vi "niScope Get Physical Cards.vi"(8 "error in":errorcluster, 11 "niScope in":T1={"channel cfg"=[], "sessions"=[], "multi cards"=FALSE, "channels"=0, "type"=enum."n/a", "memory [B/chn]"=0, "ext. clock [Hz]"=0.0, "samples count"=0, "use streaming"=FALSE, "proc setup"={"packet size [smpl]"=0, "current timeout [s]"=0.0, "blk2blk timeout [s]"=0.0, "event time"=timestamp(0 s since 1904-01-01), "temp sampl T [s]"=0.0, "data queue"=refnum, "stop notifier"=refnum, "proc ref"=refnum}, "sample width [B]"=0, "ranges [V]"=[], "trigger setup"={"coupling"=1, "level [V]"=0.0, "slope"=0, "mode"=enum."Immediate"}, "fs [Hz]"=0.0, "bitres [bit]"=0, "clock source"=enum."VAL_NO_SOURCE"} {"trigger setup"."level [V]" format="%.2f"; "trigger setup"."coupling" items=["AC"=0, "DC"=1, "HF Reject"=3, "LF Reject"=4, "AC Plus HF Reject"=1001]; "channel cfg"."Range [Vpk]" min=0.0; "channel cfg"."Channel" min=0}) -> (0 "error out":errorcluster, 2 "card list":T12[](array[typedef]), 3 "niScope out":T1={"channel cfg"=[], "sessions"=[], "multi cards"=FALSE, "channels"=0, "type"=enum."n/a", "memory [B/chn]"=0, "ext. clock [Hz]"=0.0, "samples count"=0, "use streaming"=FALSE, "proc setup"={"packet size [smpl]"=0, "current timeout [s]"=0.0, "blk2blk timeout [s]"=0.0, "event time"=timestamp(0 s since 1904-01-01), "temp sampl T [s]"=0.0, "data queue"=refnum, "stop notifier"=refnum, "proc ref"=refnum}, "sample width [B]"=0, "ranges [V]"=[], "trigger setup"={"coupling"=1, "level [V]"=0.0, "slope"=0, "mode"=enum."Immediate"}, "fs [Hz]"=0.0, "bitres [bit]"=0, "clock source"=enum."VAL_NO_SOURCE"} {"trigger setup"."level [V]" format="%.2f"; "trigger setup"."coupling" items=["AC"=0, "DC"=1, "HF Reject"=3, "LF Reject"=4, "AC Plus HF Reject"=1001]; "channel cfg"."Range [Vpk]" min=0.0; "channel cfg"."Channel" min=0})   [LabVIEW 2013, in "niScope Virtual Digitizer.lvlib"]
doc: "Scans through virtual channels list and builds list of physical channels for each unique address (device)."
uses:
  niScope Physical Cards.ctl
  niScope Session.ctl
  niScope Virtual Channel Config.ctl
  niScope Virtual Channel Mode.ctl
  niScope Virtual Channel Input Z.ctl
  niScope Virtual Channel Coupling.ctl
  niScope Type.ctl
  niScope Digitizing Process Options.ctl
  niScope Data Packet.ctl
  niScope Trigger Setup.ctl
  <instrlib>/niScope/Controls/niScope trigger coupling.ctl
  <instrlib>/niScope/Controls/niScope trigger slope.ctl
  niScope Reference Clock.ctl
  <vilib>/Utility/error.llb/Error Cluster From Error Code.vi
  <vilib>/ErrorRing/Error Ring.xnode
  niScope Virtual Digitizer.lvlib
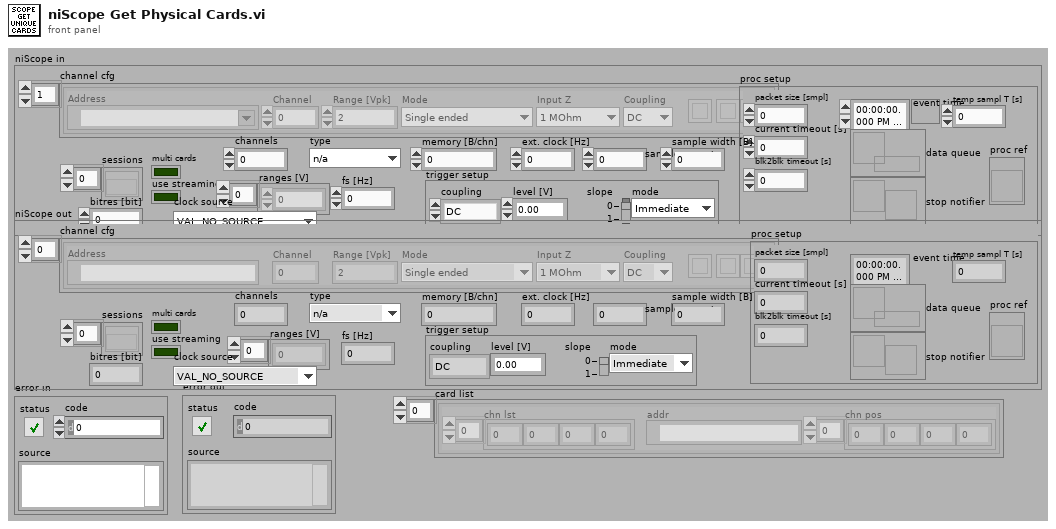
[diagram p1: front panel]
types:
  T1 = typedef "niScope Virtual Digitizer.lvlib/niScope Session.ctl" = cluster{"channel cfg":T2[], "sessions":refnum<k20>[], "multi cards":bool, "channels":i32, "type":T6, "memory [B/chn]":i32, "ext. clock [Hz]":dbl, "samples count":i64, "use streaming":bool, "proc setup":T7, "sample width [B]":i32, "ranges [V]":dbl[], "trigger setup":T8, "fs [Hz]":dbl, "bitres [bit]":i32, "clock source":T11}
  T2 = typedef "niScope Virtual Digitizer.lvlib/niScope Virtual Channel Config.ctl" = cluster{"Address":refnum<k15>, "Channel":i32, "Mode":T3, "Input Z":T4, "Coupling":T5, "Range [Vpk]":dbl, "btn clr":bool, "btn up":bool, "btn down":bool}
  T3 = typedef "niScope Virtual Digitizer.lvlib/niScope Virtual Channel Mode.ctl" = enum16{"Single ended", "Unbal. differential", "Differential"}
  T4 = typedef "niScope Virtual Digitizer.lvlib/niScope Virtual Channel Input Z.ctl" = enum16{"1 MOhm", "50 Ohm"}
  T5 = typedef "niScope Virtual Digitizer.lvlib/niScope Virtual Channel Coupling.ctl" = enum16{"AC", "DC", "GND"}
  T6 = typedef "niScope Virtual Digitizer.lvlib/niScope Type.ctl" = enum16{"n/a", "5922"}
  T7 = typedef "niScope Virtual Digitizer.lvlib/niScope Digitizing Process Options.ctl" = cluster{"packet size [smpl]":i64, "current timeout [s]":dbl, "blk2blk timeout [s]":dbl, "event time":timestamp, "temp sampl T [s]":dbl, "data queue":refnum<queue>, "stop notifier":refnum<notifier>, "proc ref":refnum<vi>}
  T8 = typedef "niScope Virtual Digitizer.lvlib/niScope Trigger Setup.ctl" = cluster{"coupling":T9, "level [V]":dbl, "slope":T10, "mode":enum16{"Immediate", "External", "Level"}}
  T9 = typedef "niScope trigger coupling.ctl" = u16
  T10 = typedef "niScope trigger slope.ctl" = i32
  T11 = typedef "niScope Virtual Digitizer.lvlib/niScope Reference Clock.ctl" = enum16{"VAL_NO_SOURCE", "VAL_CLK_IN", "VAL_PXI_CLOCK", "VAL_EXTERNAL"}
  T12 = typedef "niScope Virtual Digitizer.lvlib/niScope Physical Cards.ctl" = cluster{"chn lst":i32[], "addr":refnum<k15>, "chn pos":i32[]}
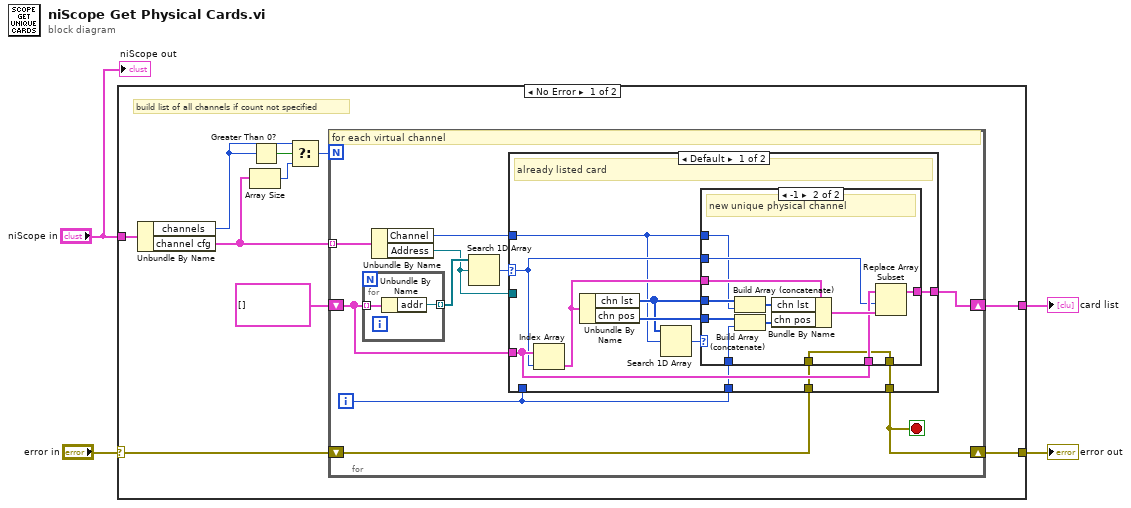
[diagram p0: block diagram]
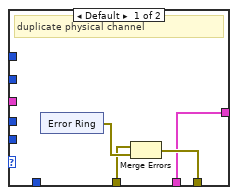
[diagram p2: hidden frame]
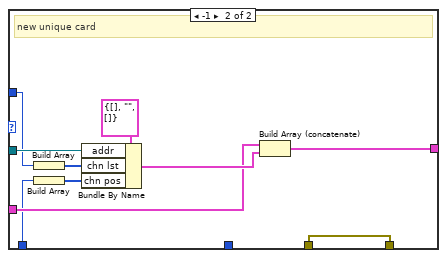
[diagram p3: hidden frame]
diagram:
  n1 = case shown="No Error" "error in" {
    selector: "error in" -> [w8 w69]
    tunnel: "niScope in" -> [w9 _]
    tunnel: [w7 _] -> w3
    tunnel: [w5 w69] -> w2
    frame No Error {
      # "build list of all channels if count not specified"
      n2 = Unbundle By Name(w9) -> ("channels"=w11:i32, "channel cfg"=w10:T2[])
      n3 = Array Size(array=w10) -> (size(s)=w12:i32)
      n4 = Greater Than 0?(x=w11) -> (x > 0?=w13:bool)
      n5 = Select(t=w11, s=w13, f=w12) -> (s? t:f=w14:i32)
      n6 = for {
        N: w14 -> [_]
        shift-right: [w21] -> w7
        shift-left: T12[] [] ("card list") -> [w22]
        tunnel: w10 -> [w19] mode=indexing
        shift-right: [w15] -> w5
        shift-left: w8 -> [w16]
        i -> [w20]
        stop <- w15 stop-if-true
        # "for each virtual channel"
        n7 = for {
          tunnel: w22 -> [w26] mode=indexing
          tunnel: [w25] -> w23 mode=indexing
          n8 = Unbundle By Name(w26) -> ("addr"=w25:refnum<k15>)
        }
        n9 = Unbundle By Name(w19) -> ("Channel"=w18:i32, "Address"=w17:refnum<k15>)
        n10 = Search 1D Array(1D array=w23, element=w17) -> (index of element=w24:i32)  [unwired: 1 in]
        n11 = case shown="Default" w24 {
          selector: w24 -> [w35 _]
          tunnel: w17 -> [_ w68]
          tunnel: [w34 w64] -> w21
          tunnel: w22 -> [w36 w65]
          tunnel: w18 -> [w30 w63]
          tunnel: w20 -> [w32 _]
          tunnel: w20 -> [_ w61]
          tunnel: w16 -> [w28 w60]
          tunnel: [w27 w60] -> w15
          frame Default {
            # "already listed card"
            n12 = Index Array(array=w36, index=w35) -> (element=w37:T12)
            n13 = Unbundle By Name(w37) -> ("chn lst"=w31:i32[], "chn pos"=w33:i32[])
            n14 = Search 1D Array(1D array=w31, element=w30) -> (index of element=w29:i32)  [unwired: 1 in]
            n15 = case shown="-1" w29 {
              tunnel: w37 -> [_ w57]
              tunnel: w36 -> [w38 w55]
              tunnel: w35 -> [_ w54]
              tunnel: [w38 w53] -> w34
              tunnel: w33 -> [_ w52]
              tunnel: w32 -> [_ w50]
              tunnel: w31 -> [_ w49]
              tunnel: w30 -> [_ w48]
              tunnel: w28 -> [w40 w47]
              tunnel: [w39 w47] -> w27
              frame Default {
                # "duplicate physical channel"
                n16 = xnode "Error Ring"() -> ("error out"=w41:errorcluster)
                n17 = Merge Errors(w40, w41) -> (w39:errorcluster)
              }
              frame -1 {
                # "new unique physical channel"
                n18 = Build Array (concatenate)(w49, w48) -> (w58:i32[])
                n19 = Build Array (concatenate)(w52, w50) -> (w51:i32[])
                n20 = Bundle By Name(cluster=w57, "chn lst"=w58, "chn pos"=w51) -> (w56:T12)
                n21 = Replace Array Subset(array=w55, new element=w56, index=w54) -> (w53:T12[])
              }
            }
          }
          frame -1 {
            # "new unique card"
            n22 = Build Array(w63) -> (w67:i32[])
            n23 = Build Array(w61) -> (w62:i32[])
            n24 = Bundle By Name(cluster=T12 {"chn lst"=[], "addr"="", "chn pos"=[]} ("Cluster"), "addr"=w68, "chn lst"=w67, "chn pos"=w62) -> (w66:T12)
            n25 = Build Array (concatenate)(w65, w66) -> (w64:T12[])
          }
        }
      }
    }
    frame Error {
    }
  }
  "card list" <- w3
  "error out" <- w2
  "niScope out" <- "niScope in"
